vi "UI_(02)_Unlock_UI.vi"(0 "All UI references in":T24, 2 "Settings cluster in":T3={"Defaults"={"Default User"=0.0, "VISA Resource Name "="", "Histogram parameters"={"max"=300.0, "min"=0.0, "# bins"=10, "threshold"=8.0, "thr. type"=enum."higher accepted"}}, "Recording and saving"={"Researcher name"="", "Name prefix"="", "Data post-processing"={"Filter type"=enum."Savitzky-Golay", "Length"=31, "Order"=3}, "Stop at"=0.0, "\"Stop at\" enabled"=FALSE, "Default save folder path"=path "", "Acquisition FPS"=enum."Max"}, "Geometry"={"Sensor board size"=enum."", "Bridge swap"=FALSE, "Twisted neck"=FALSE, "Bridge H. offset"=0.0, "Bridge V. offset"=0.0, "Magnets orientation"=0.0, "Cage type"=0, "Cage parameters"={"Round"=variant(i16 0), "Square"=variant(u16 0), "Donut-maze"=variant(u16 0), "T-maze"=variant(u8 0), "Sociability-maze"=variant(u8 0)}}, "IO parameters"={"IO general config."=0, "IO 1 configuration"=0, "IO 2 configuration"=0, "IO 3 configuration"=0, "IO 4 configuration"=0, "Activate ext. RS-232"=0, "IO inversion config."=0, "Sync capability"=1}, "Conditions presets array"=[{"Enabled"=FALSE, "Name"="", "Specifier(s)"=[], "Response"={"Response type"=enum."Air puff", "TTL port"=enum."Port 1", "TTL pulse length, ms"=0.0}, "Has been set"=FALSE}, {"Enabled"=FALSE, "Name"="", "Specifier(s)"=[], "Response"={"Response type"=enum."Air puff", "TTL port"=enum."Port 1", "TTL pulse length, ms"=0.0}, "Has been set"=FALSE}, {"Enabled"=FALSE, "Name"="", "Specifier(s)"=[], "Response"={"Response type"=enum."Air puff", "TTL port"=enum."Port 1", "TTL pulse length, ms"=0.0}, "Has been set"=FALSE}, {"Enabled"=FALSE, "Name"="", "Specifier(s)"=[], "Response"={"Response type"=enum."Air puff", "TTL port"=enum."Port 1", "TTL pulse length, ms"=0.0}, "Has been set"=FALSE}, {"Enabled"=FALSE, "Name"="", "Specifier(s)"=[], "Response"={"Response type"=enum."Air puff", "TTL port"=enum."Port 1", "TTL pulse length, ms"=0.0}, "Has been set"=FALSE}, {"Enabled"=FALSE, "Name"="", "Specifier(s)"=[], "Response"={"Response type"=enum."Air puff", "TTL port"=enum."Port 1", "TTL pulse length, ms"=0.0}, "Has been set"=FALSE}, {"Enabled"=FALSE, "Name"="", "Specifier(s)"=[], "Response"={"Response type"=enum."Air puff", "TTL port"=enum."Port 1", "TTL pulse length, ms"=0.0}, "Has been set"=FALSE}, {"Enabled"=FALSE, "Name"="", "Specifier(s)"=[], "Response"={"Response type"=enum."Air puff", "TTL port"=enum."Port 1", "TTL pulse length, ms"=0.0}, "Has been set"=FALSE}, {"Enabled"=FALSE, "Name"="", "Specifier(s)"=[], "Response"={"Response type"=enum."Air puff", "TTL port"=enum."Port 1", "TTL pulse length, ms"=0.0}, "Has been set"=FALSE}, {"Enabled"=FALSE, "Name"="", "Specifier(s)"=[], "Response"={"Response type"=enum."Air puff", "TTL port"=enum."Port 1", "TTL pulse length, ms"=0.0}, "Has been set"=FALSE}, {"Enabled"=FALSE, "Name"="", "Specifier(s)"=[], "Response"={"Response type"=enum."Air puff", "TTL port"=enum."Port 1", "TTL pulse length, ms"=0.0}, "Has been set"=FALSE}, {"Enabled"=FALSE, "Name"="", "Specifier(s)"=[], "Response"={"Response type"=enum."Air puff", "TTL port"=enum."Port 1", "TTL pulse length, ms"=0.0}, "Has been set"=FALSE}, {"Enabled"=FALSE, "Name"="", "Specifier(s)"=[], "Response"={"Response type"=enum."Air puff", "TTL port"=enum."Port 1", "TTL pulse length, ms"=0.0}, "Has been set"=FALSE}, {"Enabled"=FALSE, "Name"="", "Specifier(s)"=[], "Response"={"Response type"=enum."Air puff", "TTL port"=enum."Port 1", "TTL pulse length, ms"=0.0}, "Has been set"=FALSE}], "Calibration parameters"={"Timing calibration sw/hw"=1.0, "True FPS"=80.0, "True frame time, s"=80.0, "Disp. calibration info"=[]}} {"Calibration parameters"."True frame time, s" format="%.10g"; "Calibration parameters"."Disp. calibration info"."Speed, µl per ms" format="%.3g"; "Calibration parameters"."True FPS" format="%.10g"; "Calibration parameters"."Timing calibration sw/hw" format="%.10g"; "Conditions presets array"."Specifier(s)"."Validity criteria(s)"."Validity value" min=0.0 step=0.1 format="%.2g"; "Conditions presets array"."Specifier(s)"."Value" step=1.0 format="%#.2g"; "Recording and saving"."Data post-processing"."Order" min=3 max=11 step=2; "Recording and saving"."Data post-processing"."Length" min=5 max=301 step=2; "Geometry"."Cage type" items=["Round", "Square", "Donut-maze", "T-maze", "Sociability maze", ""]}, 3 "error in (no error)":errorcluster, 4 "Optional Information in":variant) -> (6 "error out":errorcluster)   [LabVIEW 2018, in "Tracker Main.lvlib"]
uses:
  Tracker Main.lvlib
  Common/Typedefs/CTL_All_UI_References_2.ctl
  Common/Typedefs/CTL_Panes_and_VIs_References.ctl
  Common/Typedefs/CTL_Indicators_References_2.ctl
  Common/Typedefs/CTL_Controls_References_2.ctl
  SubVi's/Controls/CTL_Histogram_Properties.ctl
  <vilib>/Utility/miscctls.llb/LVRangeTypeDef.ctl
  Common/Typedefs/CTL_Settings_cluster_2.ctl
  SubVi's/Controls/CTL_Histogram_parameters.ctl
  SubVi's/Controls/CTL_Filter_selector.ctl
  SubVi's/Controls/CTL_Acquisition_speed_selector.ctl
  Common/Typedefs/CTL_Segmented_plot_parameters_2.ctl
  Cage Diagram/Typedefs/CTL_Cage_type.ctl
  SubVi's/Controls/CTL_Cage_all_segmentation_params_set.ctl
  SubVi's/Controls/CTL_IO_params_cluster.ctl
  SubVi's/Controls/CTL_Conditions_Array.ctl
  SubVi's/Controls/CTL_Conditions_Cluster.ctl
  SubVi's/Controls/CTL_Condition_type.ctl
  SubVi's/Controls/CTL_Comparison_type.ctl
  SubVi's/Controls/CTL_Validity_check_criteria.ctl
  SubVi's/Controls/CTL_Response_info.ctl
  SubVi's/Controls/CTL_Condition_response_type.ctl
  SubVi's/Controls/CTL_Reponse_port_info.ctl
  SubVi's/Controls/CTL_Calibration_parameters.ctl
  SubVi's/Controls/CTL_Dispenser_calibration_info.ctl
  <vilib>/Utility/miscctls.llb/LVPointTypeDef.ctl
  HW Init Outcome check Argument--cluster.ctl
  HW Interaction/Public API/Typedefs/CTL_Sensor_board_type_(size).ctl
  Common/Typedefs/CTL_Segmented_plot_parameters_2_(round_d1).ctl
  Common/Typedefs/CTL_IO_Ports_activity_indicator.ctl
  <vilib>/Utility/error.llb/Error Cluster From Error Code.vi
  <vilib>/ErrorRing/Error Ring.xnode
  Common_Resources.lvlib
  HW Interaction/HW Interaction.lvlib
  Cage Diagram/Cage Diagram.lvlib
panel:
  out "Controls References":T1
  out "Indicators References":T2
  in  "Histogram initialization cluster":T21={"X Scale.Range"={"Minimum"=0.0, "Maximum"=13.0, "Increment"=1.0, "Minor Increment"=1.0, "Start"=0.0}, "Caption.Text"="Zone preference (normalized)", "X Scale.Offset and Multiplier:Multiplier"=1.0, "X Scale.Offset and Multiplier:Offset"=0.0, "X Scale.Scale Fit"=2, "X Scale.Display Format:Precision"=0, "Y Scale.Mapping Mode"=0, "Zones preference empty initialized array"=[0, 0, 0, 0, 0, 0, 0, 0, 0, 0, 0, 0, 0, 0], "Plot.Fill/Point Color"=15790320}
  out "Panes references":T23
  out "Controls references params":string[][](array[string])
  out "Indicators references params":string[][](array[string])
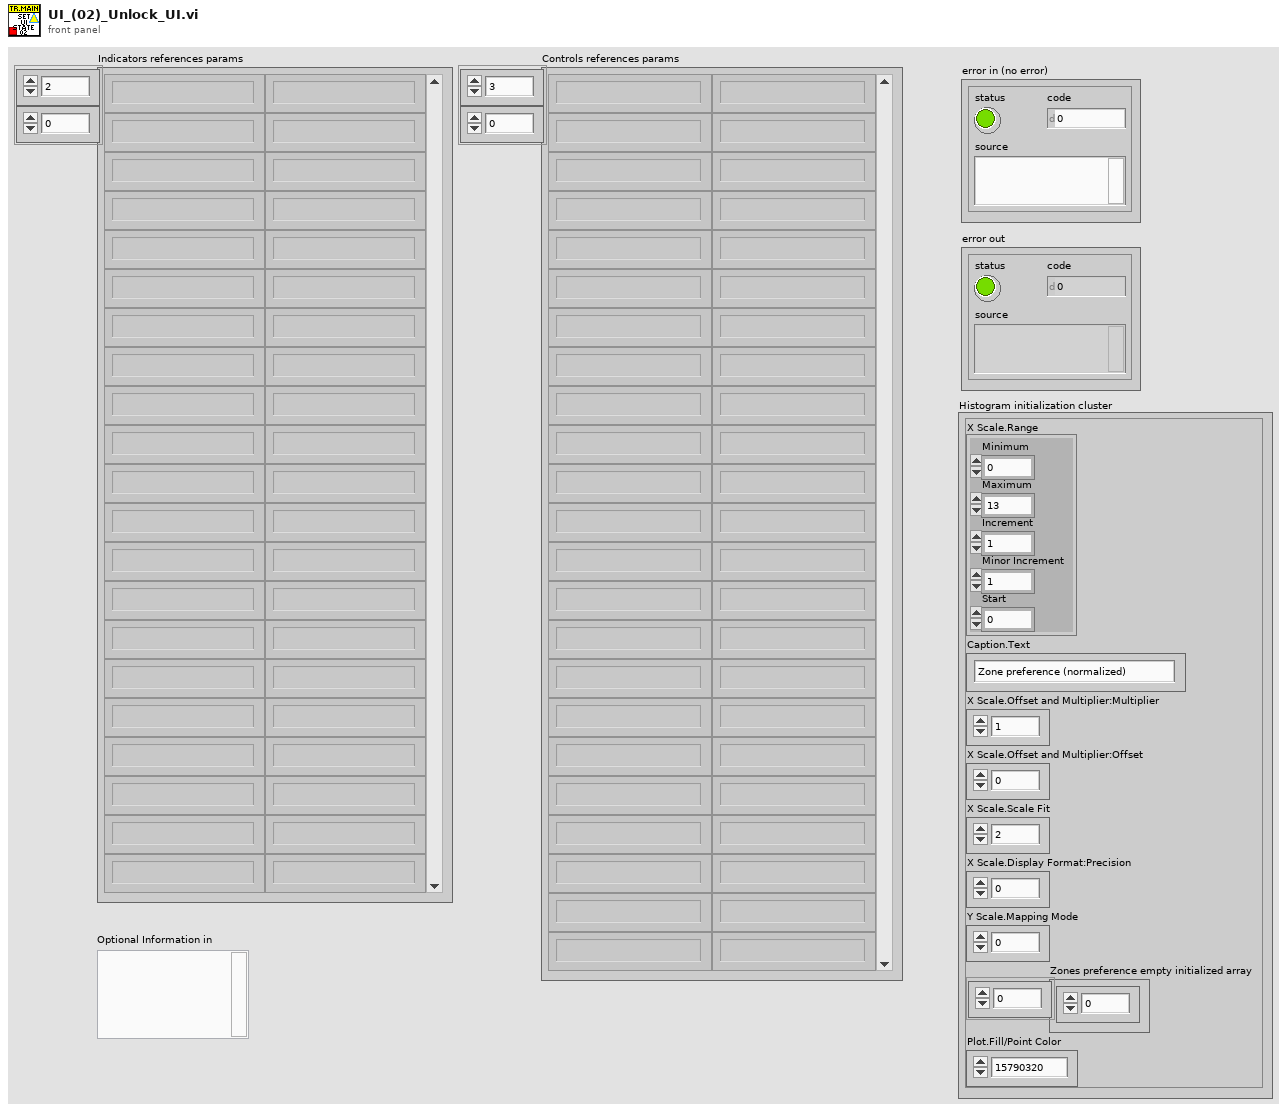
[diagram p1: front panel]
types:
  T1 = typedef "Common_Resources.lvlib/CTL_Controls_References_2.ctl" = cluster{"Timeline":refnum<vi>, "Play/Pause":refnum<vi>, "Record/Stop":refnum<vi>, "Exact time pos.":refnum<vi>, "Add Reward":refnum<vi>, "Modify Reward":refnum<vi>, "Remove Reward":refnum<vi>, "Show zones":refnum<vi>, "Show magnets":refnum<vi>, "Rainbow (time)":refnum<vi>, "Rainbow (speed)":refnum<vi>, "Show heatmap":refnum<vi>, "Show full track":refnum<vi>, "Playback speed":refnum<vi>, "Trace, s":refnum<vi>, "Set/Rec and Analyse Tab":refnum<vi>, "Reward and stimulation":refnum<vi>, "Speed threshold":refnum<vi>, "Multiplyer of chart RX":refnum<vi>, "Reset barplot":refnum<vi>, "Open File":refnum<vi>, "Start over":refnum<vi>}
  T2 = typedef "Common_Resources.lvlib/CTL_Indicators_References_2.ctl" = cluster{"HW info":refnum<vi>, "Port":refnum<vi>, "Cage size":refnum<vi>, "Current zone":refnum<vi>, "Current Time":refnum<vi>, "Since track start":refnum<vi>, "Key_pressed":refnum<vi>, "Status":refnum<vi>, "Status History":refnum<vi>, "IO status":refnum<vi>, "Ports Activity":refnum<vi>, "Active rules":refnum<vi>, "Histograms":refnum<vi>, "Mouse speed":refnum<vi>, "Mouse speed, mm/s":refnum<vi>, "Average speed, mm/s":refnum<vi>, "Run distance, m":refnum<vi>, "Running, perc. of time":refnum<vi>, "CPU load":refnum<vi>, "Diagram ref":refnum<vi>}
  T3 = typedef "Common_Resources.lvlib/CTL_Settings_cluster_2.ctl" = cluster{"Defaults":cluster{"Default User":dbl, "VISA Resource Name ":string, "Histogram parameters":T4}, "Recording and saving":cluster{"Researcher name":string, "Name prefix":string, "Data post-processing":T5, "Stop at":dbl, "\"Stop at\" enabled":bool, "Default save folder path":path, "Acquisition FPS":T6}, "Geometry":T7, "IO parameters":T10, "Conditions presets array":T11, "Calibration parameters":T19}
  T4 = typedef "Common_Resources.lvlib/CTL_Histogram_parameters.ctl" = cluster{"max":dbl, "min":dbl, "# bins":i32, "threshold":dbl, "thr. type":enum16{"higher accepted", "lower accepted"}}
  T5 = typedef "Common_Resources.lvlib/CTL_Filter_selector.ctl" = cluster{"Filter type":enum16{"None", "Savitzky-Golay"}, "Length":i32, "Order":i32}
  T6 = typedef "Common_Resources.lvlib/CTL_Acquisition_speed_selector.ctl" = enum16{"Max", "Optimal", "Eco"}
  T7 = typedef "Common_Resources.lvlib/CTL_Segmented_plot_parameters_2.ctl" = cluster{"Sensor board size":enum16{"", "Large"}, "Bridge swap":bool, "Twisted neck":bool, "Bridge H. offset":sgl, "Bridge V. offset":sgl, "Magnets orientation":sgl, "Cage type":T8, "Cage parameters":T9}
  T8 = typedef "Cage Diagram.lvlib/CTL_Cage_type.ctl" = u16
  T9 = typedef "Common_Resources.lvlib/CTL_Cage_all_segmentation_params_set.ctl" = cluster{"Round":variant, "Square":variant, "Donut-maze":variant, "T-maze":variant, "Sociability-maze":variant}
  T10 = typedef "Common_Resources.lvlib/CTL_IO_params_cluster.ctl" = cluster{"IO general config.":u16, "IO 1 configuration":u16, "IO 2 configuration":u16, "IO 3 configuration":u16, "IO 4 configuration":u16, "Activate ext. RS-232":u16, "IO inversion config.":u16, "Sync capability":u8}
  T11 = typedef "Common_Resources.lvlib/CTL_Conditions_Array.ctl" = T12[]
  T12 = typedef "Common_Resources.lvlib/CTL_Conditions_Cluster.ctl" = cluster{"Enabled":bool, "Name":string, "Specifier(s)":cluster{"Specifier enabled":bool, "Condition type":T13, "Comparison type":T14, "Value":dbl, "Validity criteria(s)":cluster{"V. check enabled":bool, "Criteria":T15, "Validity value":dbl}[]}[], "Response":T16, "Has been set":bool}
  T13 = typedef "Common_Resources.lvlib/CTL_Condition_type.ctl" = enum16{"Speed", "Zone", "Angle to wall"}
  T14 = typedef "Common_Resources.lvlib/CTL_Comparison_type.ctl" = enum16{"Less", "Less or Equal", "Equal", "Greater or Equal", "Greater", "Not Equal"}
  T15 = typedef "Common_Resources.lvlib/CTL_Validity_check_criteria.ctl" = enum16{"Running bout (seconds)", "Running bout (meters)"}
  T16 = typedef "Common_Resources.lvlib/CTL_Response_info.ctl" = cluster{"Response type":T17, "TTL port":T18, "TTL pulse length, ms":dbl}
  T17 = typedef "Common_Resources.lvlib/CTL_Condition_response_type.ctl" = enum16{"None", "Air puff", "Liquid reward", "TTL pulse", "TTL pulse (ubr)", "TTL signal"}
  T18 = typedef "Common_Resources.lvlib/CTL_Reponse_port_info.ctl" = enum16{"Port 1", "Port 2", "Port 3", "Port 4"}
  T19 = typedef "Common_Resources.lvlib/CTL_Calibration_parameters.ctl" = cluster{"Timing calibration sw/hw":dbl, "True FPS":dbl, "True frame time, s":dbl, "Disp. calibration info":T20}
  T20 = typedef "Common_Resources.lvlib/CTL_Dispenser_calibration_info.ctl" = cluster{"Channel":u8, "Speed, µl per ms":dbl}[]
  T21 = typedef "Common_Resources.lvlib/CTL_Histogram_Properties.ctl" = cluster{"X Scale.Range":T22, "Caption.Text":string, "X Scale.Offset and Multiplier:Multiplier":dbl, "X Scale.Offset and Multiplier:Offset":dbl, "X Scale.Scale Fit":u8, "X Scale.Display Format:Precision":u8, "Y Scale.Mapping Mode":u8, "Zones preference empty initialized array":i32[], "Plot.Fill/Point Color":u32}
  T22 = typedef "LVRangeTypeDef.ctl" = cluster{"Minimum":dbl, "Maximum":dbl, "Increment":dbl, "Minor Increment":dbl, "Start":dbl}
  T23 = typedef "Common_Resources.lvlib/CTL_Panes_and_VIs_References.ctl" = cluster{"Pane":refnum<vi>, "This VI":refnum<vi>, "Menu":refnum<k9>}
  T24 = typedef "Common_Resources.lvlib/CTL_All_UI_References_2.ctl" = cluster{"Service references":T23, "Indicators References":T2, "Controls References":T1}
  T25 = typedef "Tracker Main.lvlib/HW Init Outcome check Argument--cluster.ctl" = cluster{"Outcome":cluster{"HW Init OK?":bool, "Sensor board type":T26, "FW Version":string, "HW set FPS":dbl, "Sync capability":u8}}
  T26 = typedef "HW Interaction.lvlib/CTL_Sensor_board_type_(size).ctl" = enum16{"Small", "Large"}
  T27 = typedef "LVPointTypeDef.ctl" = cluster{"Horizontal":i16, "Vertical":i16}
  T28 = typedef "Common_Resources.lvlib/CTL_Segmented_plot_parameters_2_(round_d1).ctl" = cluster{"Cage diameter, mm":u16, "Starting angle BORDER":i16, "Starting angle MIDFIELD":i16, "Radius, mm MIDFIELD":u16, "Radius, mm CENTER":u16, "N segments BORDER":u8, "N segments MIDFIELD":u8, "R-gap, mm":sgl}
  T29 = typedef "Common_Resources.lvlib/CTL_IO_Ports_activity_indicator.ctl" = cluster{"IO1 act":bool, "IO2 act":bool, "IO3 act":bool, "IO4 act":bool}
  T30 = cluster{"01":bool, "02":bool, "03":bool, "04":bool, "05":bool, "06":bool, "07":bool, "08":bool, "09":bool}
  T31 = enum8{"Enabled", "Disabled", "Disabled and Grayed Out"}
  T32 = enum32{"Page Enabled", "Page Disabled", "Page Disabled & Grayed"}
  T33 = cluster{"Slider":dbl, "Slider":dbl, "Slider":dbl}
  T34 = typedef "Common_Resources.lvlib/CTL_IO_status_indicator_2.ctl" = cluster{"IO1":bool, "IO2":bool, "IO3":bool, "IO4":bool, "St1":bool, "St2":bool, "St3":bool, "St4":bool, "Ext1":bool, "Ext2":bool, "Ext3":bool, "Ext4":bool, "Syn1":bool, "Syn2":bool, "Syn3":bool, "Syn4":bool}
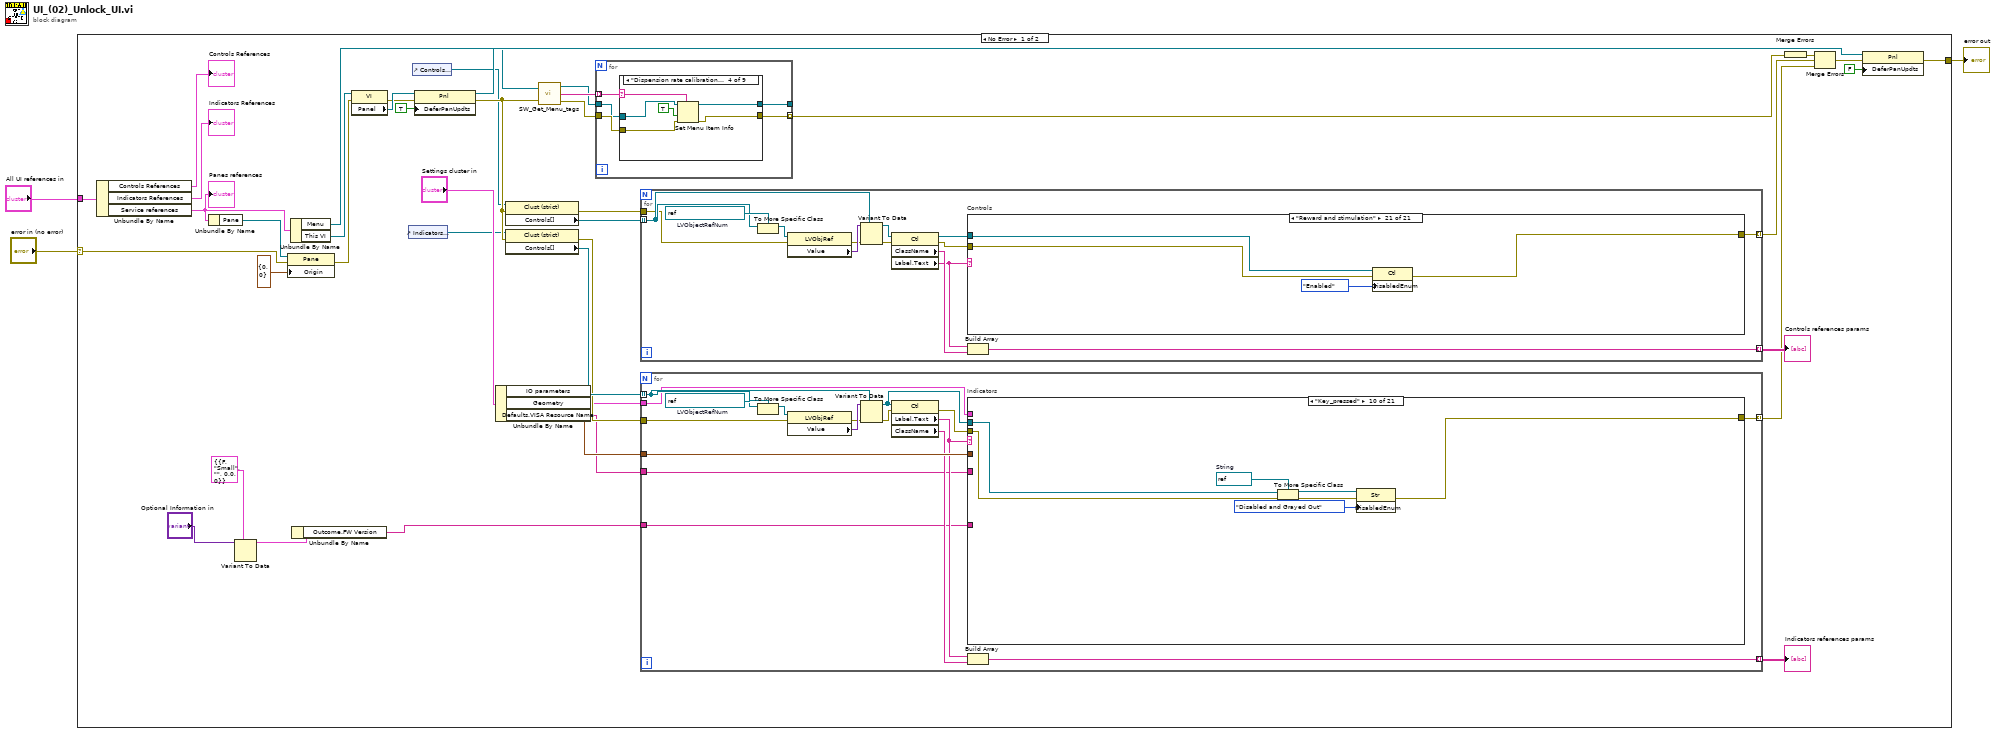
[diagram p0: block diagram]
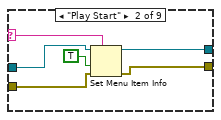
[diagram p3: hidden frame]
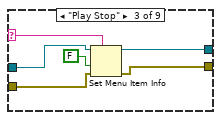
[diagram p4: hidden frame]
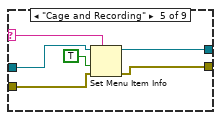
[diagram p5: hidden frame]
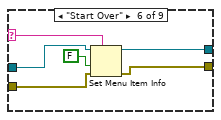
[diagram p6: hidden frame]
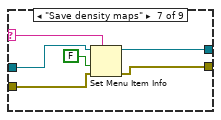
[diagram p7: hidden frame]
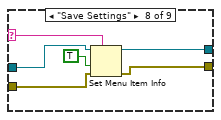
[diagram p8: hidden frame]
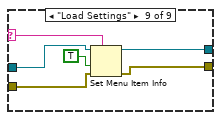
[diagram p9: hidden frame]
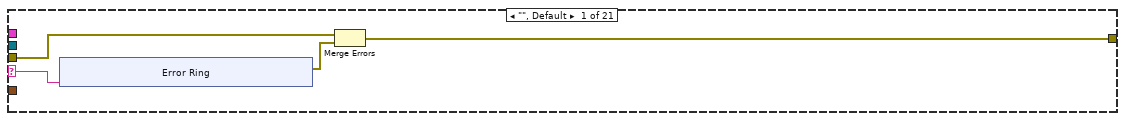
[diagram p10: hidden frame]
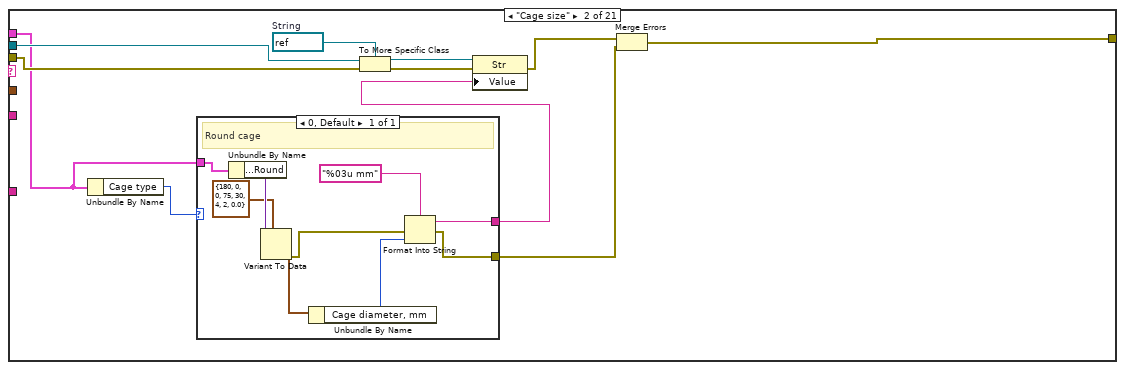
[diagram p11: hidden frame]
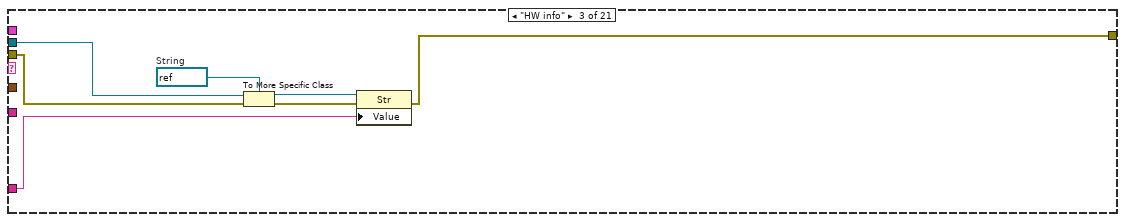
[diagram p12: hidden frame]
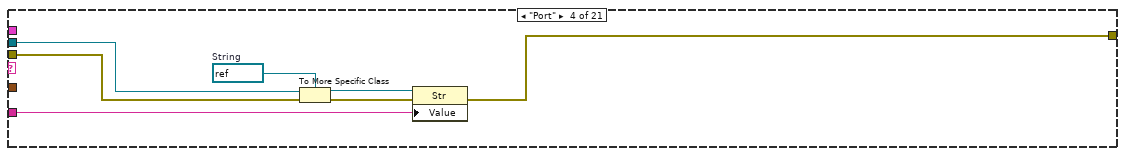
[diagram p13: hidden frame]
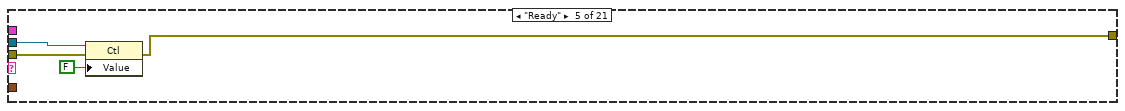
[diagram p14: hidden frame]
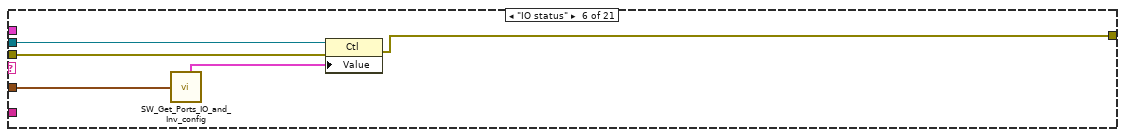
[diagram p15: hidden frame]
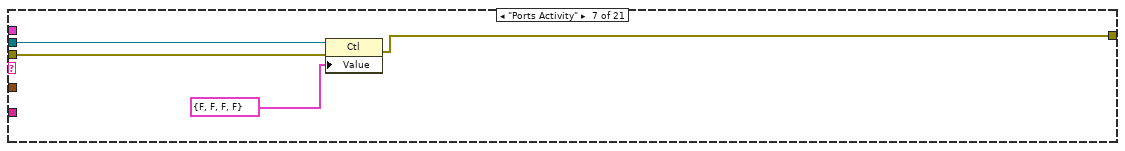
[diagram p16: hidden frame]
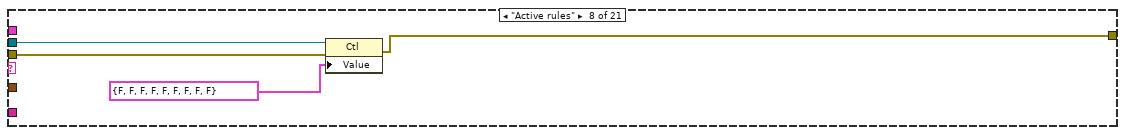
[diagram p17: hidden frame]
diagram:
  n1 = case shown="No Error" "error in (no error)" {
    selector: "error in (no error)" -> [w9 w432]
    tunnel: "All UI references in" -> [w44 _]
    tunnel: [w29 w432] -> w2
    frame No Error {
      n2 = Unbundle By Name(w44) -> ("Controls References"=→"Controls References":T1, "Indicators References"=→"Indicators References":T2, "Service references"=w14:T23)
      "Panes references" <- w14
      n3 = Unbundle By Name(w14) -> ("Pane"=w26:refnum<vi>)
      n4 = Variant To Data(type=T25 {"Outcome"={"HW Init OK?"=FALSE, "Sensor board type"=enum."Small", "FW Version"="", "HW set FPS"=0.0, "Sync capability"=0}} ("HW Init Outcome check Argument"), Variant="Optional Information in") -> (data=w6:T25)  [unwired: 1 in, 1 out]
      n5 = property class="Pane"(reference=w26, error in=w9, "Origin"=T27 {"Horizontal"=0, "Vertical"=0}) -> (error out=w25:errorcluster)  [unwired: 1 out]
      n6 = Unbundle By Name(w14) -> ("Menu"=w23:refnum<k9>, "This VI"=w37:refnum<vi>)
      n7 = Unbundle By Name(w6) -> ("Outcome.FW Version"=w4:string)
      n8 = property class="VI"(reference=w37, error in=w25) -> (error out=w30:errorcluster, "Panel"=w39:refnum<vi>)  [unwired: 1 out]
      n9 = control-ref of="Indicators References"() -> (w12:refnum<vi>)
      n10 = control-ref of="Controls References"() -> (w10:refnum<vi>)
      n11 = property class="Pnl"(reference=w39, error in=w30, "DeferPanUpdts"=TRUE ("Defer Panel Updates")) -> (reference out=w31:refnum<vi>, error out=w22:errorcluster)
      n12 = Unbundle By Name("Settings cluster in") -> ("IO parameters"=w27:T10, "Geometry"=w15:T7, "Defaults.VISA Resource Name"=w5:string)
      n13 = property class="Clust (strict)"(reference=w10, error in=w22) -> (error out=w36:errorcluster, "Controls[]"=w43:refnum<vi>[])  [unwired: 1 out]
      n14 = property class="Clust (strict)"(reference=w12, error in=w22) -> (error out=w35:errorcluster, "Controls[]"=w42:refnum<vi>[])  [unwired: 1 out]
      n15 = call "SW_Get_Menu_tags.vi"("Menu ref in"=w23, "error in (no error)"=w22) -> ("Menu ref out"=w19:refnum<k9>, "(Sub)menu tags"=w21:string[], "error out"=w20:errorcluster)
      n16 = for {
        tunnel: w21 -> [w49] mode=indexing
        tunnel: w20 -> [w48]
        tunnel: [w47] -> w18 mode=indexing
        tunnel: [w46] -> _
        tunnel: w19 -> [w45]
        n17 = case shown="\"Dispension rate calibration\", \"Fix broken track\", \"I/O Configuration\", \"Timings calibration\", \"Tools\"" w49 {
          selector: w49 -> [_ w57 w63 w69 w75 w81 w87 w93 w99]
          tunnel: w48 -> [w51 w55 w61 w67 w73 w79 w85 w91 w97]
          tunnel: [w51 w54 w60 w66 w72 w78 w84 w90 w96] -> w47
          tunnel: [w50 w53 w59 w65 w71 w77 w83 w89 w95] -> w46
          tunnel: w45 -> [w50 w52 w58 w64 w70 w76 w82 w88 w94]
          frame "", Default {
          }
          frame "Play Start" {
            n18 = Set Menu Item Info(7:w57, 8:w55, 9:TRUE ("enabled"), 11:w52) -> (0:w54:errorcluster, 3:w53:refnum<k9>)  [unwired: 3 in]
          }
          frame "Play Stop" {
            n19 = Set Menu Item Info(7:w63, 8:w61, 9:FALSE ("enabled"), 11:w58) -> (0:w60:errorcluster, 3:w59:refnum<k9>)  [unwired: 3 in]
          }
          frame "Dispension rate calibration", "Fix broken track", "I/O Configuration", "Timings calibration", "Tools" {
            n20 = Set Menu Item Info(7:w69, 8:w67, 9:TRUE ("enabled"), 11:w64) -> (0:w66:errorcluster, 3:w65:refnum<k9>)  [unwired: 3 in]
          }
          frame "Cage and Recording" {
            n21 = Set Menu Item Info(7:w75, 8:w73, 9:TRUE ("enabled"), 11:w70) -> (0:w72:errorcluster, 3:w71:refnum<k9>)  [unwired: 3 in]
          }
          frame "Start Over" {
            n22 = Set Menu Item Info(7:w81, 8:w79, 9:FALSE ("enabled"), 11:w76) -> (0:w78:errorcluster, 3:w77:refnum<k9>)  [unwired: 3 in]
          }
          frame "Save density maps" {
            n23 = Set Menu Item Info(7:w87, 8:w85, 9:FALSE ("enabled"), 11:w82) -> (0:w84:errorcluster, 3:w83:refnum<k9>)  [unwired: 3 in]
          }
          frame "Save Settings" {
            n24 = Set Menu Item Info(7:w93, 8:w91, 9:TRUE ("enabled"), 11:w88) -> (0:w90:errorcluster, 3:w89:refnum<k9>)  [unwired: 3 in]
          }
          frame "Load Settings" {
            n25 = Set Menu Item Info(7:w99, 8:w97, 9:TRUE ("enabled"), 11:w94) -> (0:w96:errorcluster, 3:w95:refnum<k9>)  [unwired: 3 in]
          }
        }
      }
      n26 = for {
        tunnel: w43 -> [w245] mode=indexing
        tunnel: [w242] -> w40 mode=indexing
        tunnel: w36 -> [w241]
        tunnel: [w237] -> w28 mode=indexing
        w247 = refnum<vi> refnum  # LVObjectRefNum
        n27 = To More Specific Class(target class=w247, reference=w245) -> (specific class reference=w248:refnum<vi>)  [unwired: 1 in, 1 out]
        n28 = property class="LVObjRef"(reference=w248, error in=w241) -> (error out=w240:errorcluster, "Value"=w246:variant)  [unwired: 1 out]
        n29 = Variant To Data(error in=w240, type=w245, Variant=w246) -> (data=w244:refnum<vi>, error out=w239:errorcluster)
        n30 = property class="Ctl"(reference=w244, error in=w239) -> (reference out=w235:refnum<vi>, error out=w236:errorcluster, "ClassName"=w243:string, "Label.Text"=w238:string)
        n31 = case "Controls" shown="\"Reward and stimulation\"" w238 {
          selector: w238 -> [w249 _ _ _ _ _ _ _ _ _ _ _ _ _ _ _ _ _ _ _ _]
          tunnel: [w251 w260 w277 w286 w294 w302 w310 w318 w326 w334 w342 w350 w358 w366 w374 w382 w389 w396 w404 w420 w428] -> w237
          tunnel: w236 -> [w252 w264 w279 w288 w296 w304 w312 w320 w328 w336 w344 w352 w360 w368 w376 w384 w391 w398 w406 w422 w429]
          tunnel: w235 -> [_ w269 w282 w291 w299 w307 w315 w323 w331 w339 w347 w355 w363 w371 w379 w387 w394 w401 w409 w425 w430]
          frame "", Default {
            n32 = xnode "Error Ring"("parameter 0"=w249) -> ("error out"=w250:errorcluster)
            n33 = Merge Errors(w252, w250) -> (w251:errorcluster)
          }
          frame "Set/Rec and Analyse Tab" {
            w266 = refnum<vi> refnum  # TabControl
            n34 = To More Specific Class(target class=w266, reference=w269, error in=w264) -> (specific class reference=w267:refnum<vi>, error out=w263:errorcluster)
            n35 = property class="TabCtl"(reference=w267, error in=w263, "Value"=enum32{"Settings", "Recording and Analysis"}."Settings") -> (error out=w262:errorcluster, "Pages"=w265:refnum<vi>[])  [unwired: 1 out]
            n36 = for {
              tunnel: w265 -> [w272] mode=indexing
              tunnel: w262 -> [w271]
              tunnel: [w270] -> w261 mode=indexing
              n37 = property class="Page"(reference=w272, error in=w271, "PageEnb"=T32."Page Enabled" ("Page Enabled State")) -> (error out=w270:errorcluster)  [unwired: 1 out]
            }
            n38 = Merge Errors(w261) -> (w260:errorcluster)
          }
          frame "Record/Stop" {
            w281 = refnum<vi> refnum  # Boolean
            n39 = To More Specific Class(target class=w281, reference=w282, error in=w279) -> (specific class reference=w280:refnum<vi>, error out=w278:errorcluster)
            n40 = property class="Bool"(reference=w280, error in=w278, "Value"=FALSE, "DisabledEnum"=T31."Disabled and Grayed Out" ("Disabled"), "Visible"=TRUE) -> (error out=w277:errorcluster)  [unwired: 1 out]
          }
          frame "Start over" {
            w290 = refnum<vi> refnum  # Boolean
            n41 = To More Specific Class(target class=w290, reference=w291, error in=w288) -> (specific class reference=w289:refnum<vi>, error out=w287:errorcluster)
            n42 = property class="Bool"(reference=w289, error in=w287, "Value"=FALSE, "DisabledEnum"=T31."Disabled and Grayed Out" ("Disabled"), "Visible"=TRUE) -> (error out=w286:errorcluster)  [unwired: 1 out]
          }
          frame "Reset barplot" {
            w298 = refnum<vi> refnum  # Boolean
            n43 = To More Specific Class(target class=w298, reference=w299, error in=w296) -> (specific class reference=w297:refnum<vi>, error out=w295:errorcluster)
            n44 = property class="Bool"(reference=w297, error in=w295, "Value"=FALSE, "DisabledEnum"=T31."Disabled and Grayed Out" ("Disabled")) -> (error out=w294:errorcluster)  [unwired: 1 out]
          }
          frame "Multiplyer of chart RX" {
            w306 = refnum<vi> refnum  # Slide
            n45 = To More Specific Class(target class=w306, reference=w307, error in=w304) -> (specific class reference=w305:refnum<vi>, error out=w303:errorcluster)
            n46 = property class="Slide"(reference=w305, error in=w303, "Value"=u8 1, "DisabledEnum"=T31."Disabled and Grayed Out" ("Disabled")) -> (error out=w302:errorcluster)  [unwired: 1 out]
          }
          frame "Show zones" {
            w314 = refnum<vi> refnum  # Boolean
            n47 = To More Specific Class(target class=w314, reference=w315, error in=w312) -> (specific class reference=w313:refnum<vi>, error out=w311:errorcluster)
            n48 = property class="Bool"(reference=w313, error in=w311, "Value"=TRUE, "DisabledEnum"=T31."Enabled" ("Disabled")) -> (error out=w310:errorcluster)  [unwired: 1 out]
          }
          frame "Show magnets" {
            w322 = refnum<vi> refnum  # Boolean
            n49 = To More Specific Class(target class=w322, reference=w323, error in=w320) -> (specific class reference=w321:refnum<vi>, error out=w319:errorcluster)
            n50 = property class="Bool"(reference=w321, error in=w319, "Value"=FALSE, "DisabledEnum"=T31."Disabled and Grayed Out" ("Disabled")) -> (error out=w318:errorcluster)  [unwired: 1 out]
          }
          frame "Rainbow (speed)", "Rainbow (time)" {
            w330 = refnum<vi> refnum  # Boolean
            n51 = To More Specific Class(target class=w330, reference=w331, error in=w328) -> (specific class reference=w329:refnum<vi>, error out=w327:errorcluster)
            n52 = property class="Bool"(reference=w329, error in=w327, "Value"=FALSE, "DisabledEnum"=T31."Disabled and Grayed Out" ("Disabled")) -> (error out=w326:errorcluster)  [unwired: 1 out]
          }
          frame "Add Reward" {
            w338 = refnum<vi> refnum  # Boolean
            n53 = To More Specific Class(target class=w338, reference=w339, error in=w336) -> (specific class reference=w337:refnum<vi>, error out=w335:errorcluster)
            n54 = property class="Bool"(reference=w337, error in=w335, "Value"=FALSE, "DisabledEnum"=T31."Enabled" ("Disabled")) -> (error out=w334:errorcluster)  [unwired: 1 out]
          }
          frame "Modify Reward", "Remove Reward" {
            w346 = refnum<vi> refnum  # Boolean
            n55 = To More Specific Class(target class=w346, reference=w347, error in=w344) -> (specific class reference=w345:refnum<vi>, error out=w343:errorcluster)
            n56 = property class="Bool"(reference=w345, error in=w343, "Value"=FALSE, "DisabledEnum"=T31."Disabled and Grayed Out" ("Disabled")) -> (error out=w342:errorcluster)  [unwired: 1 out]
          }
          frame "Show heatmap" {
            w354 = refnum<vi> refnum  # Boolean
            n57 = To More Specific Class(target class=w354, reference=w355, error in=w352) -> (specific class reference=w353:refnum<vi>, error out=w351:errorcluster)
            n58 = property class="Bool"(reference=w353, error in=w351, "Value"=FALSE, "DisabledEnum"=T31."Disabled and Grayed Out" ("Disabled")) -> (error out=w350:errorcluster)  [unwired: 1 out]
          }
          frame "Show full track" {
            w362 = refnum<vi> refnum  # Boolean
            n59 = To More Specific Class(target class=w362, reference=w363, error in=w360) -> (specific class reference=w361:refnum<vi>, error out=w359:errorcluster)
            n60 = property class="Bool"(reference=w361, error in=w359, "Value"=FALSE, "DisabledEnum"=T31."Disabled and Grayed Out" ("Disabled")) -> (error out=w358:errorcluster)  [unwired: 1 out]
          }
          frame "Open File" {
            w370 = refnum<vi> refnum  # Boolean
            n61 = To More Specific Class(target class=w370, reference=w371, error in=w368) -> (specific class reference=w369:refnum<vi>, error out=w367:errorcluster)
            n62 = property class="Bool"(reference=w369, error in=w367, "Value"=FALSE, "DisabledEnum"=T31."Enabled" ("Disabled")) -> (error out=w366:errorcluster)  [unwired: 1 out]
          }
          frame "Play/Pause" {
            w378 = refnum<vi> refnum  # Boolean
            n63 = To More Specific Class(target class=w378, reference=w379, error in=w376) -> (specific class reference=w377:refnum<vi>, error out=w375:errorcluster)
            n64 = property class="Bool"(reference=w377, error in=w375, "Value"=FALSE, "DisabledEnum"=T31."Enabled" ("Disabled")) -> (error out=w374:errorcluster)  [unwired: 1 out]
          }
          frame "Trace, s" {
            w386 = refnum<vi> refnum  # Slide
            n65 = To More Specific Class(target class=w386, reference=w387, error in=w384) -> (specific class reference=w385:refnum<vi>, error out=w383:errorcluster)
            n66 = property class="Slide"(reference=w385, error in=w383, "Value"=u8 5, "DisabledEnum"=T31."Disabled and Grayed Out" ("Disabled")) -> (error out=w382:errorcluster)  [unwired: 1 out]
          }
          frame "Speed threshold" {
            w393 = refnum<vi> refnum  # Digital
            n67 = To More Specific Class(target class=w393, reference=w394, error in=w391) -> (specific class reference=w392:refnum<vi>, error out=w390:errorcluster)
            n68 = property class="DigNum"(reference=w392, error in=w390, "DisabledEnum"=T31."Disabled and Grayed Out" ("Disabled")) -> (error out=w389:errorcluster)  [unwired: 1 out]
          }
          frame "Exact time pos." {
            w400 = refnum<vi> refnum  # Digital
            n69 = To More Specific Class(target class=w400, reference=w401, error in=w398) -> (specific class reference=w399:refnum<vi>, error out=w397:errorcluster)
            n70 = property class="DigNum"(reference=w399, error in=w397, "DisabledEnum"=T31."Disabled and Grayed Out" ("Disabled")) -> (error out=w396:errorcluster)  [unwired: 1 out]
          }
          frame "Playback speed" {
            w408 = refnum<vi> refnum  # Ring
            n71 = To More Specific Class(target class=w408, reference=w409, error in=w406) -> (specific class reference=w407:refnum<vi>, error out=w405:errorcluster)
            n72 = property class="Ring"(reference=w407, error in=w405, "Value"=u8 120, "DisabledEnum"=T31."Disabled and Grayed Out" ("Disabled")) -> (error out=w404:errorcluster)  [unwired: 1 out]
          }
          frame "Timeline" {
            w411 = 0.0 ("Slider")
            w424 = refnum<vi> refnum  # Slide
            n73 = To More Specific Class(target class=w424, reference=w425, error in=w422) -> (specific class reference=w423:refnum<vi>, error out=w421:errorcluster)
            n74 = Bundle(cluster=T33 {"Slider"=0.0, "Slider"=0.0, "Slider"=0.0} ("Timeline"), "Slider"=w411, "Slider"=0.001, "Slider"=w411) -> (w417:T33)
            n75 = To Variant(anything=w417) -> (Variant=w416:variant)
            n76 = property class="Slide"(reference=w423, error in=w421, "Value"=w416, "DisabledEnum"=T31."Disabled and Grayed Out" ("Disabled"), "Scale.Minimum"=0.0 ("Scale.Range:Minimum"), "Scale.Maximum"=60.0 ("Scale.Range:Maximum"), "Scale.RngStart"=0.0 ("Scale.Range:Start")) -> (error out=w420:errorcluster, "DigDisps[]"=w410:refnum<vi>[])  [unwired: 1 out]
            n77 = for {
              tunnel: w410 -> [w427] mode=indexing
              n78 = property class="DigNum"(reference=w427, "Visible"=FALSE) -> ()  [unwired: 1 in, 2 out]
            }
          }
          frame "Reward and stimulation" {
            n79 = property class="Ctl"(reference=w430, error in=w429, "DisabledEnum"=T31."Enabled" ("Disabled")) -> (error out=w428:errorcluster)  [unwired: 1 out]
          }
        }
        n80 = Build Array(w238, w243) -> (w242:string[])
      }
      "Controls references params" <- w40
      n81 = for {
        tunnel: w42 -> [w113] mode=indexing
        tunnel: [w103] -> w41 mode=indexing
        tunnel: w35 -> [w111]
        tunnel: [w107] -> w34 mode=indexing
        tunnel: w27 -> [w106]
        tunnel: w15 -> [w102]
        tunnel: w4 -> [w101]
        tunnel: w5 -> [w100]
        w115 = refnum<vi> refnum  # LVObjectRefNum
        n82 = To More Specific Class(target class=w115, reference=w113) -> (specific class reference=w116:refnum<vi>)  [unwired: 1 in, 1 out]
        n83 = property class="LVObjRef"(reference=w116, error in=w111) -> (error out=w110:errorcluster, "Value"=w114:variant)  [unwired: 1 out]
        n84 = Variant To Data(error in=w110, type=w113, Variant=w114) -> (data=w112:refnum<vi>, error out=w109:errorcluster)
        n85 = property class="Ctl"(reference=w112, error in=w109) -> (error out=w108:errorcluster, "Label.Text"=w105:string, "ClassName"=w104:string)  [unwired: 1 out]
        n86 = case "Indicators" shown="\"Key_pressed\"" w105 {
          selector: w105 -> [w117 _ _ _ _ _ _ _ _ _ _ _ _ _ _ _ _ _ _ _ _]
          tunnel: w112 -> [_ w134 w154 w158 w165 w167 w172 w176 _ w180 _ _ w193 w198 w203 w208 w213 w218 w225 w232 _]
          tunnel: w108 -> [w120 w135 w153 w157 w164 w168 w173 w177 w179 w183 w187 w188 w192 w197 w202 w207 w212 w217 w224 w228 w234]
          tunnel: [w119 w130 w148 w155 w163 w170 w174 w178 w179 w181 w187 w188 w191 w196 w201 w206 w211 w216 w220 w231 w234] -> w107
          tunnel: w106 -> [_ _ _ _ _ w169 _ _ _ _ _ _ _ _ _ _ _ _ _ _ _]
          tunnel: w102 -> [_ w131 _ _ _ _ _ _ _ _ _ _ _ _ _ _ _ _ w219 _ _]
          tunnel: w101 -> [_ _ w149 _ _ _ _ _ _ _ _ _ _ _ _ _ _ _ _ _ _]
          tunnel: w100 -> [_ _ _ w156 _ _ _ _ _ _ _ _ _ _ _ _ _ _ _ _ _]
          frame "", Default {
            n87 = xnode "Error Ring"("parameter 0"=w117) -> ("error out"=w118:errorcluster)
            n88 = Merge Errors(w120, w118) -> (w119:errorcluster)
          }
          frame "Cage size" {
            w138 = refnum<vi> refnum  # String
            n89 = Unbundle By Name(w131) -> ("Cage type"=w132:T8)
            n90 = case shown="0, Default" w132 {
              tunnel: w131 -> [w147]
              tunnel: [w141] -> w129
              tunnel: [w139] -> w128
              frame 0, Default {
                # "Round cage"
                n91 = Unbundle By Name(w147) -> ("Cage parameters.Round"=w146:variant)
                n92 = Variant To Data(type=T28 {"Cage diameter, mm"=180, "Starting angle BORDER"=0, "Starting angle MIDFIELD"=0, "Radius, mm MIDFIELD"=75, "Radius, mm CENTER"=30, "N segments BORDER"=4, "N segments MIDFIELD"=2, "R-gap, mm"=0.0} ("Radial segmentation parameters"), Variant=w146) -> (data=w144:T28, error out=w142:errorcluster)  [unwired: 1 in]
                n93 = Unbundle By Name(w144) -> ("Cage diameter, mm"=w143:u16)
                n94 = Format Into String(format string="%03u mm", error in=w142, w143) -> (resulting string=w139:string, error out=w141:errorcluster)  [unwired: 1 in]
              }
            }
            n95 = To More Specific Class(target class=w138, reference=w134, error in=w135) -> (specific class reference=w136:refnum<vi>, error out=w137:errorcluster)
            n96 = property class="Str"(reference=w136, error in=w137, "Value"=w128) -> (error out=w133:errorcluster)  [unwired: 1 out]
            n97 = Merge Errors(w133, w129) -> (w130:errorcluster)
          }
          frame "HW info" {
            w152 = refnum<vi> refnum  # String
            n98 = To More Specific Class(target class=w152, reference=w154, error in=w153) -> (specific class reference=w150:refnum<vi>, error out=w151:errorcluster)
            n99 = property class="Str"(reference=w150, error in=w151, "Value"=w149) -> (error out=w148:errorcluster)  [unwired: 1 out]
          }
          frame "Port" {
            w161 = refnum<vi> refnum  # String
            n100 = To More Specific Class(target class=w161, reference=w158, error in=w157) -> (specific class reference=w159:refnum<vi>, error out=w160:errorcluster)
            n101 = property class="Str"(reference=w159, error in=w160, "Value"=w156) -> (error out=w155:errorcluster)  [unwired: 1 out]
          }
          frame "Ready" {
            n102 = property class="Ctl"(reference=w165, error in=w164, "Value"=FALSE) -> (error out=w163:errorcluster)  [unwired: 1 out]
          }
          frame "IO status" {
            n103 = call "SW_Get_Ports_IO_and_Inv_config.vi"("IO parameters cluster input"=w169) -> ("IO status indicator 2"=w166:T34)  [unwired: 4 out]
            n104 = property class="Ctl"(reference=w167, error in=w168, "Value"=w166) -> (error out=w170:errorcluster)  [unwired: 1 out]
          }
          frame "Ports Activity" {
            n105 = property class="Ctl"(reference=w172, error in=w173, "Value"=T29 {"IO1 act"=FALSE, "IO2 act"=FALSE, "IO3 act"=FALSE, "IO4 act"=FALSE} ("Ports Activity")) -> (error out=w174:errorcluster)  [unwired: 1 out]
          }
          frame "Active rules" {
            n106 = property class="Ctl"(reference=w176, error in=w177, "Value"=T30 {"01"=FALSE, "02"=FALSE, "03"=FALSE, "04"=FALSE, "05"=FALSE, "06"=FALSE, "07"=FALSE, "08"=FALSE, "09"=FALSE} ("Active rules")) -> (error out=w178:errorcluster)  [unwired: 1 out]
          }
          frame "Current Time" {
          }
          frame "Key_pressed" {
            w186 = refnum<vi> refnum  # String
            n107 = To More Specific Class(target class=w186, reference=w180, error in=w183) -> (specific class reference=w184:refnum<vi>, error out=w185:errorcluster)
            n108 = property class="Str"(reference=w184, error in=w185, "DisabledEnum"=T31."Disabled and Grayed Out" ("Disabled")) -> (error out=w181:errorcluster)  [unwired: 1 out]
          }
          frame "Status" {
          }
          frame "Status History" {
          }
          frame "Since track start" {
            n109 = property class="Ctl"(reference=w193, error in=w192, "Value"=0.0, "DisabledEnum"=T31."Disabled and Grayed Out" ("Disabled")) -> (error out=w191:errorcluster)  [unwired: 1 out]
          }
          frame "Mouse speed" {
            n110 = property class="Ctl"(reference=w198, error in=w197, "Value"=waveform(dbl)[] [] ("History Data"), "DisabledEnum"=T31."Disabled and Grayed Out" ("Disabled")) -> (error out=w196:errorcluster)  [unwired: 1 out]
          }
          frame "Mouse speed, mm/s" {
            n111 = property class="Ctl"(reference=w203, error in=w202, "Value"=0.0, "DisabledEnum"=T31."Disabled and Grayed Out" ("Disabled")) -> (error out=w201:errorcluster)  [unwired: 1 out]
          }
          frame "Average speed, mm/s" {
            n112 = property class="Ctl"(reference=w208, error in=w207, "Value"=0.0, "DisabledEnum"=T31."Disabled and Grayed Out" ("Disabled")) -> (error out=w206:errorcluster)  [unwired: 1 out]
          }
          frame "CPU load" {
            n113 = property class="Ctl"(reference=w213, error in=w212, "Value"=0.0, "DisabledEnum"=T31."Disabled" ("Disabled")) -> (error out=w211:errorcluster)  [unwired: 1 out]
          }
          frame "Run distance, m", "Running, perc. of time" {
            n114 = property class="Ctl"(reference=w218, error in=w217, "Value"=0.0, "DisabledEnum"=T31."Disabled and Grayed Out" ("Disabled")) -> (error out=w216:errorcluster)  [unwired: 1 out]
          }
          frame "Current zone" {
            w223 = refnum<vi> refnum  # Cluster
            n115 = To More Specific Class(target class=w223, reference=w225, error in=w224) -> (specific class reference=w221:refnum<vi>, error out=w222:errorcluster)
            n116 = call "UI_update_Zone_indicator_params_(univ).vi"("error in (no error)"=w222, "Geometry"=w219, "Zone indicator ref. in"=w221) -> ("error out"=w220:errorcluster)  [unwired: 7 in, 1 out]
          }
          frame "Histograms" {
            w229 = refnum<vi> refnum  # XYGraph
            n117 = disable-structure shown="Disabled" {
              frame Disabled {
                n118 = Unbundle By Name("Histogram initialization cluster") -> ()  [unwired: 9 out]
              }
              frame Enabled {
              }
            }
            n119 = To More Specific Class(target class=w229, reference=w232, error in=w228) -> (specific class reference=w230:refnum<vi>, error out=w227:errorcluster)
            n120 = property class="XYGraph"(reference=w230, error in=w227, "DisabledEnum"=T31."Disabled and Grayed Out" ("Disabled")) -> (error out=w231:errorcluster)  [unwired: 1 out]
          }
          frame "Diagram" {
          }
        }
        n121 = Build Array(w105, w104) -> (w103:string[])
      }
      "Indicators references params" <- w41
      n122 = Merge Errors(w18) -> (w17:errorcluster)
      n123 = Merge Errors(w17, w28, w34) -> (w33:errorcluster)
      n124 = property class="Pnl"(reference=w31, error in=w33, "DeferPanUpdts"=FALSE ("Defer Panel Updates")) -> (error out=w29:errorcluster)  [unwired: 1 out]
    }
    frame Error {
    }
  }
  "error out" <- w2
